vi "GraphSetting Get AllParam (XY).vi"(8 "エラー入力（エラーなし）":errorcluster, 11 "XYグラフref(in)":refnum<vi>) -> (0 "エラー出力":errorcluster, 3 "クラスタ":cluster{"外観(out)":T1, T2[], T2[], T4[]} {"?"."Yスケール" items=["振幅1234", "振幅 2", "振幅 33"]; "?"."Xスケール" items=["XX"]; "?"."プロット補間" max=5 step=1; "?"."ポイントスタイル" max=16 step=1; "?"."太さ" max=5 step=1; "?"."ラインスタイル" max=4 step=1})   [LabVIEW 2016]
uses:
  TypeDef/GraphSetting Appearance.ctl
  GraphSetting Scale.ctl
  TypeDef/GraphSetting DisplayFormatType.ctl
  TypeDef/GraphSetting Plot.ctl
  TypeDef/GraphSetting Command.ctl
panel:
  # "スケールのスタイルとカラー"
  # "スケール係数"
  # "スケールのスタイルとカラー"
  # "スケールのスタイルとカラー"
  # "スケール係数"
  # "スケールのスタイルとカラー"
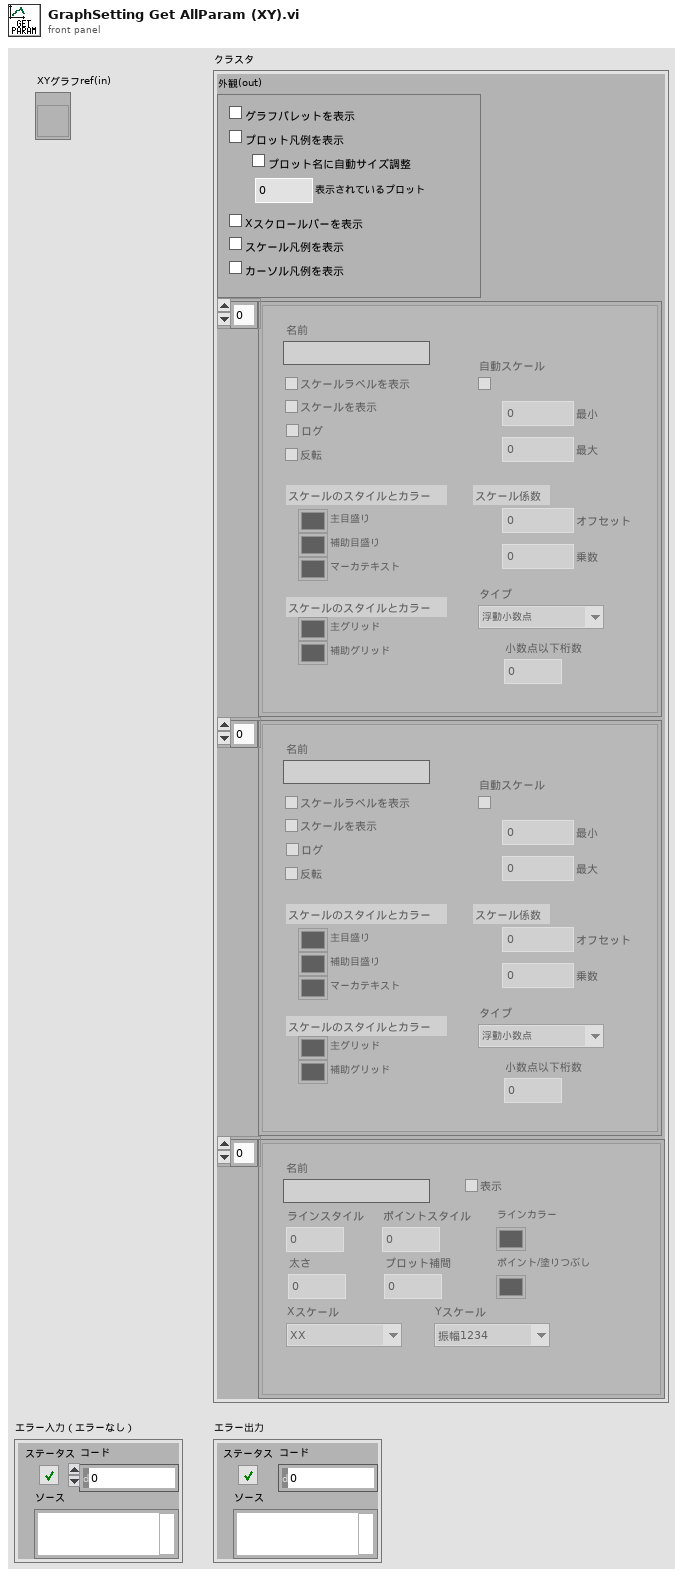
[diagram p1: front panel]
types:
  T1 = typedef "GraphSetting Appearance.ctl" = cluster{"グラフパレットを表示":bool, "プロット凡例を表示":bool, "プロット名に自動サイズ調整":bool, "表示されているプロット":u32, "Xスクロールバーを表示":bool, "スケール凡例を表示":bool, "カーソル凡例を表示":bool}
  T2 = typedef "GraphSetting Scale.ctl" = cluster{"名前":string, "スケールラベルを表示":bool, "スケールを表示":bool, "ログ":bool, "反転":bool, "自動スケール":bool, "最小":dbl, "最大":dbl, "オフセット":dbl, "乗数":dbl, "主目盛り":u32, "補助目盛り":u32, "マーカテキスト":u32, "主グリッド":u32, "補助グリッド":u32, "タイプ":T3, "小数点以下桁数":u8}
  T3 = typedef "GraphSetting DisplayFormatType.ctl" = enum8{"浮動小数点", "科学", "工学", "バイナリ", "８進数", "１６進数", "相対時間", "時間と日時", "SI"}
  T4 = typedef "GraphSetting Plot.ctl" = cluster{"名前":string, "表示":bool, "ラインスタイル":u8, "太さ":u8, "ポイントスタイル":u8, "プロット補間":u8, "ラインカラー":u32, "ポイント/塗りつぶし":u32, "Xスケール":u16, "Yスケール":u16}
  T5 = typedef "GraphSetting Command.ctl" = enum16{"Get(ref->ctl)", "Set(ctl->ref)"}
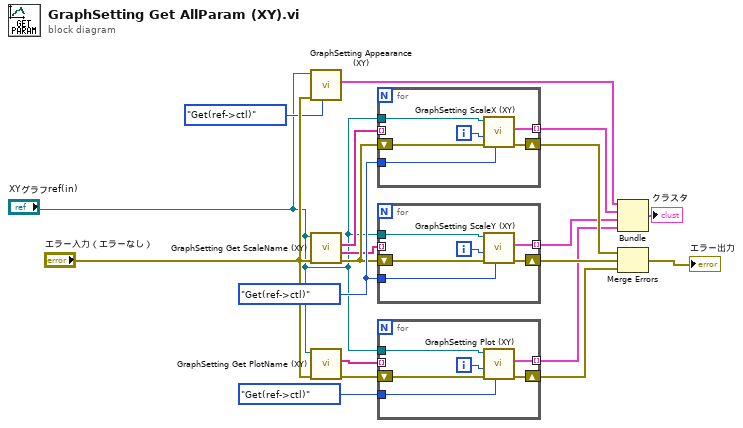
[diagram p0: block diagram]
diagram:
  w13 = GraphSetting_Command."Get(ref->ctl)" ("コマンド")
  n1 = call "GraphSetting Appearance (XY).vi"("コマンド"=GraphSetting_Command."Get(ref->ctl)", "error in (no error)"="エラー入力（エラーなし）", "XYグラフref(in)"="XYグラフref(in)") -> ("外観(out)"=w7:T1)  [unwired: 7 in, 1 out]
  n2 = call "GraphSetting Get ScaleName (XY).vi"("error in (no error)"="エラー入力（エラーなし）", "XYグラフref(in)"="XYグラフref(in)") -> ("error out"=w10:errorcluster, "Y軸名称[]"=w2:string[], "X軸名称[]"=w14:string[])  [unwired: 7 in]
  n3 = call "GraphSetting Get PlotName (XY).vi"("error in (no error)"="エラー入力（エラーなし）", "XYグラフref(in)"="XYグラフref(in)") -> ("error out"=w11:errorcluster, "プロット名称[]"=w12:string[])  [unwired: 8 in]
  n4 = for {
    tunnel: w14 -> [_] mode=indexing
    tunnel: "XYグラフref(in)" -> [w24]
    tunnel: [w23] -> w6 mode=indexing
    shift-right: [w21] -> w16
    shift-left: w10 -> [w22]
    tunnel: w13 -> [w20]
    i -> [w25]
    n5 = call "GraphSetting ScaleX (XY).vi"("コマンド"=w20, "error in (no error)"=w22, "アクティブスケール(X)"=w25, "XYグラフref(in)"=w24) -> ("error out"=w21:errorcluster, "スケール(out)"=w23:T2)  [unwired: 6 in]
  }
  n6 = for {
    tunnel: "XYグラフref(in)" -> [w30]
    tunnel: [w29] -> w5 mode=indexing
    shift-right: [w27] -> w17
    shift-left: w10 -> [w28]
    tunnel: w13 -> [w26]
    tunnel: w2 -> [_] mode=indexing
    i -> [w31]
    n7 = call "GraphSetting ScaleY (XY).vi"("コマンド"=w26, "error in (no error)"=w28, "アクティブスケールY"=w31, "XYグラフref(in)"=w30) -> ("error out"=w27:errorcluster, "スケール(out)"=w29:T2)  [unwired: 6 in]
  }
  n8 = for {
    tunnel: "XYグラフref(in)" -> [w37]
    tunnel: w12 -> [_] mode=indexing
    shift-right: [w35] -> w18
    shift-left: w11 -> [w36]
    tunnel: GraphSetting_Command."Get(ref->ctl)" ("コマンド") -> [w34]
    tunnel: [w32] -> w4 mode=indexing
    i -> [w33]
    n9 = call "GraphSetting Plot (XY).vi"("コマンド"=w34, "error in (no error)"=w36, "アクティブプロット"=w33, "XYグラフref(in)"=w37) -> ("error out"=w35:errorcluster, "プロット(out)"=w32:T4)  [unwired: 6 in]
  }
  n10 = Bundle("外観(out)"=w7, w6, w5, w4) -> (→"クラスタ":cluster{"外観(out)":T1, T2[], T2[], T4[]})  [unwired: 1 in]
  n11 = Merge Errors(w16, w17, w18) -> (→"エラー出力":errorcluster)
